vi "Add Standard Resolvers.vi"(8 "error in (no error)":errorcluster, 11 "BasicTemplater in":refnum<class "BasicTemplater.lvclass">) -> (0 "error out":errorcluster, 3 "BasicTemplater out":refnum<class "BasicTemplater.lvclass">)   [LabVIEW 2020, in "HTTP Server.lvlib" / "BasicTemplater.lvclass"]
uses:
  BasicTemplater.lvclass
  BasicTemplater.lvclass/BasicTemplater.ctl
  IncludeResolver/IncludeResolver.lvclass
  C:/dev/lv20CE/relink/lv-http-server/HTTP Server/IncludeResolver/IncludeResolver.lvclass
  C:/dev/lv20CE/relink/lv-http-server/HTTP Server/TemplateVariableResolver/TemplateValueResolver.lvclass
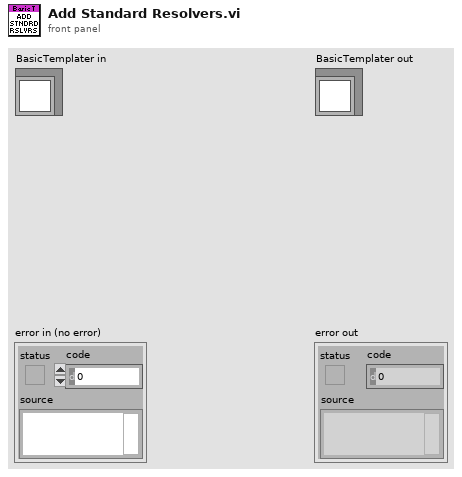
[diagram p1: front panel]
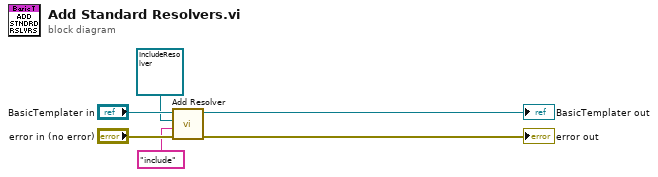
[diagram p0: block diagram]
diagram:
  n1 = call "Add Resolver.vi"("error in (no error)"="error in (no error)", "Namespace"="include", "Resolver"=refnum<class "IncludeResolver.lvclass"> refnum ("HTTP Server:IncludeResolver.lvclass"), "BasicTemplater in"="BasicTemplater in") -> ("error out"=→"error out":errorcluster, "BasicTemplater out"=→"BasicTemplater out":refnum<class "BasicTemplater.lvclass">)  [unwired: 6 in]
